vi "SimpleJoint.vi"(2 "Joint":T4={"Joint Name"="left_wheel_hinge", "type"=enum."revolute", "axis"=enum."Y"}, 3 "Child Link":T3, 4 "Parent Link":T3, 5 "origin":T5) -> (1 "Joint":T1={"Joint Name"="left_wheel_hinge", "type"=enum."revolute", "urdf "="", "Links"=[]})   [LabVIEW 2010]
uses:
  JointAttributes.ctl
  LINK.ctl
  Position.ctl
  JointTypes.ctl
  JOINT.ctl
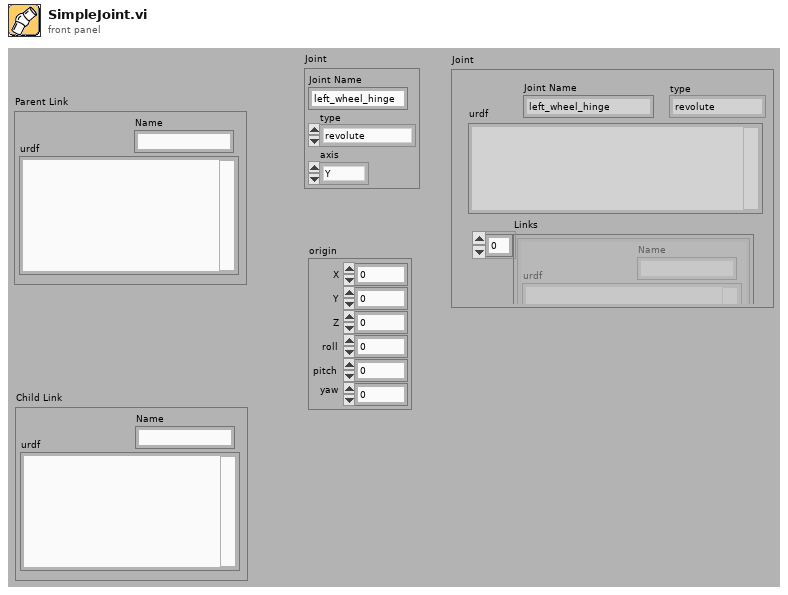
[diagram p1: front panel]
types:
  T1 = typedef "JOINT.ctl" = cluster{"Joint Name":string, "type":T2, "urdf ":string, "Links":T3[]}
  T2 = typedef "JointTypes.ctl" = enum16{"revolute", "continuous", "prismatic", "fixed", "floating", "planar"}
  T3 = typedef "LINK.ctl" = cluster{"Name":string, "urdf":string}
  T4 = cluster{"Joint Name":string, "type":T2, "axis":enum16{"X", "Y", "Z"}}
  T5 = typedef "Position.ctl" = cluster{"X":sgl, "Y":sgl, "Z":sgl, "roll":sgl, "pitch":sgl, "yaw":sgl}
  T6 = typedef "JointAttributes.ctl" = cluster{"origin":string, "parent":string, "child":string, "axis":string, "calibration":string, "dynamics":string, "mimic":string, "safety_controller":string}
  T7 = cluster{"X":sgl, "Y":sgl, "Z":sgl, "roll":sgl, "pitch":sgl, "yaw":sgl}
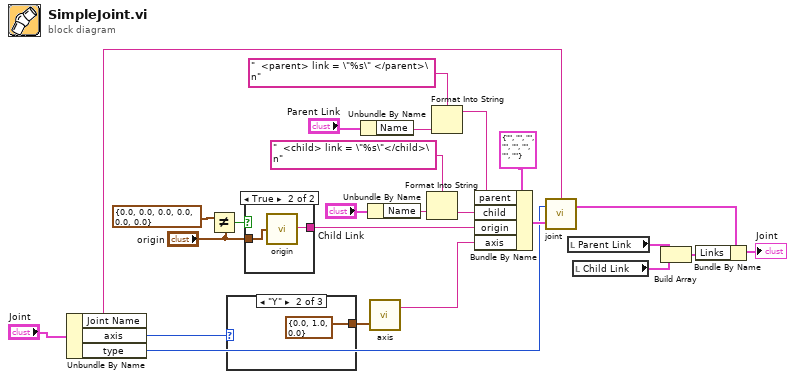
[diagram p0: block diagram]
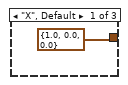
[diagram p2: hidden frame]
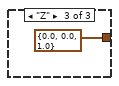
[diagram p3: hidden frame]
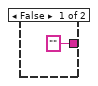
[diagram p4: hidden frame]
diagram:
  n1 = Unbundle By Name("Joint") -> ("Joint Name"=w17:string, "axis"=w16:enum16{"X", "Y", "Z"}, "type"=w6:T2)
  n2 = Not Equal?(x=T7 {"X"=0.0, "Y"=0.0, "Z"=0.0, "roll"=0.0, "pitch"=0.0, "yaw"=0.0} ("Pose of geometry"), y="origin") -> (x != y?=w20:bool)
  n3 = case shown="\"Y\"" w16 {
    tunnel: [cluster{"X":sgl, "Y":sgl, "Z":sgl} {"X"=1.0, "Y"=0.0, "Z"=0.0} ("Pose") cluster{"X":sgl, "Y":sgl, "Z":sgl} {"X"=0.0, "Y"=1.0, "Z"=0.0} ("Pose") cluster{"X":sgl, "Y":sgl, "Z":sgl} {"X"=0.0, "Y"=0.0, "Z"=1.0} ("Pose")] -> w24
    frame "X", Default {
    }
    frame "Y" {
    }
    frame "Z" {
    }
  }
  n4 = case shown="True" w20 {
    tunnel: ["" ("sdf out") w31] -> w23
    tunnel: "origin" -> [_ w30]
    frame False {
    }
    frame True {
      n5 = call "origin.vi"("origin"=w30) -> ("urdf out"=w31:string)
    }
  }
  n6 = Unbundle By Name("Parent Link") -> ("Name"=w9:string)
  n7 = Unbundle By Name("Child Link") -> ("Name"=w8:string)
  n8 = call "axis.vi"("origin"=w24) -> ("urdf out"=w25:string)  [unwired: 3 in]
  n9 = Format Into String(format string="  <child> link = \"%s\"</child>\n", w8) -> (resulting string=w11:string)  [unwired: 2 in, 1 out]
  n10 = Format Into String(format string="  <parent> link = \"%s\" </parent>\n", w9) -> (resulting string=w13:string)  [unwired: 2 in, 1 out]
  n11 = Bundle By Name(cluster=T6 {"origin"="", "parent"="", "child"="", "axis"="", "calibration"="", "dynamics"="", "mimic"="", "safety_controller"=""} ("Attributes"), "parent"=w13, "child"=w11, "origin"=w23, "axis"=w25) -> (w19:T6)
  n12 = call "joint.vi"("Attributes"=w19, "type"=w6, "Name"=w17) -> ("Joint"=w5:T1)  [unwired: 1 in]
  n13 = local read "Parent Link"() -> (w3:T3)
  n14 = local read "Child Link"() -> (w2:T3)
  n15 = Build Array(w3, w2) -> (w1:T3[])
  n16 = Bundle By Name(cluster=w5, "Links"=w1) -> (→"Joint":T1)
